vi "Convert_to_number.vi"(0 "string":string) -> (1 "offset past number":i32, 2 "Number":dbl format="%.2f")   [LabVIEW 2010]
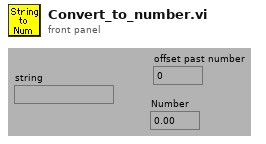
[diagram p1: front panel]
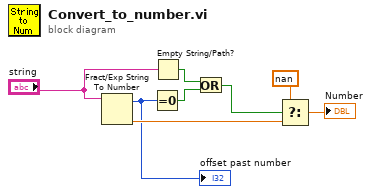
[diagram p0: block diagram]
diagram:
  n1 = Fract/Exp String To Number(string="string") -> (offset past number=w4:i32, number=w7:dbl)  [unwired: 3 out]
  "offset past number" <- w4
  n2 = Equal To 0?(x=w4) -> (x = 0?=w3:bool)
  n3 = Empty String/Path?(string/path="string") -> (empty?=w2:bool)
  n4 = Or(x=w2, y=w3) -> (x .or. y?=w1:bool)
  n5 = Select(t=nan, s=w1, f=w7) -> (s? t:f=→"Number":dbl)
